vi "Find Entity by ID.vi"(7 "Entity Type":refnum<class "Entity.lvclass">, 8 "error in (no error)":errorcluster, 9 "Entity ID":T1, 10 "Types":refnum<class "Type.lvclass">[](array[class]), 11 "Database in":refnum<class "Database Platform.lvclass">) -> (0 "error out":errorcluster, 2 "Entity":refnum<class "Entity.lvclass">, 3 "Database out":refnum<class "Database Platform.lvclass">)   [LabVIEW 2022 SP3, in "Conditum.lvlib" / "Database Platform.lvclass"]
uses:
  Database Platform.lvclass
  Entity/Entity.lvclass
  Entity ID.ctl
  Conditum.lvlib
  Columns/Type/Type.lvclass
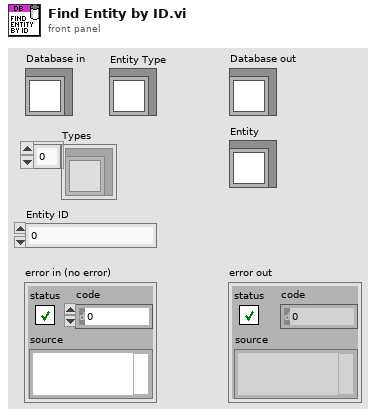
[diagram p1: front panel]
types:
  T1 = typedef "Conditum.lvlib/Entity ID.ctl" = i64
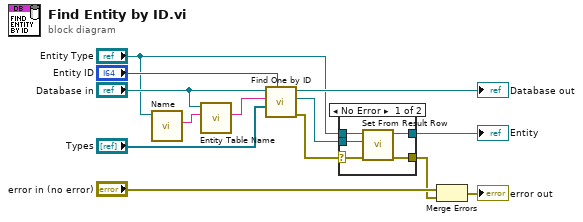
[diagram p0: block diagram]
diagram:
  n1 = call-dynamic "Name.vi"("Entity in"="Entity Type") -> ("Name"=w11:string)  [unwired: 10 in]
  n2 = call-dynamic "Entity Table Name.vi"("Entity Name"=w11, "Database in"="Database in") -> ("Table Name"=w9:string)  [unwired: 9 in]
  n3 = call-dynamic "Find One by ID.vi"("Entity ID"="Entity ID", "Entity Definition"="Types", "Table Name"=w9, "Database in"="Database in") -> ("error out"=w13:errorcluster, "Result Row"=w6:refnum<class "Result Row.lvclass">, "Database out"=→"Database out":refnum<class "Database Platform.lvclass">)  [unwired: 5 in]
  n4 = case shown="No Error" w13 {
    selector: w13 -> [w16 w19]
    tunnel: "Entity Type" -> [w18 w20]
    tunnel: w6 -> [w17 _]
    tunnel: [w15 w20] -> w5
    tunnel: [w14 w19] -> w3
    frame No Error {
      n5 = call "Set From Result Row.vi"("error in (no error)"=w16, "Result Row"=w17, "Entity in"=w18) -> ("error out"=w14:errorcluster, "Entity out"=w15:refnum<class "Entity.lvclass">)  [unwired: 7 in]
    }
    frame Error {
    }
  }
  "Entity" <- w5
  n6 = Merge Errors("error in (no error)", w3) -> (→"error out":errorcluster)
